vi "Create Keys (AO).vi"(3 "Numeric":i32) -> (1 "AO Keys":string[](array[string]))   [LabVIEW 2016, in "Transport.lvclass"]
uses:
  Transport.lvclass
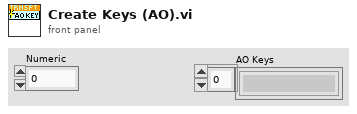
[diagram p1: front panel]
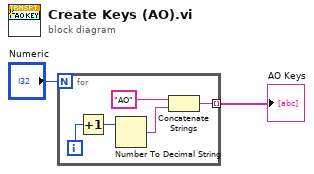
[diagram p0: block diagram]
diagram:
  n1 = for {
    N: "Numeric" -> [_]
    tunnel: [w3] -> w2 mode=indexing
    i -> [w4]
    n2 = Increment(x=w4) -> (x+1=w7:i32)
    n3 = Number To Decimal String(number=w7) -> (decimal integer string=w5:string)  [unwired: 1 in]
    n4 = Concatenate Strings("AO" ("wavenames"), w5) -> (w3:string)
  }
  "AO Keys" <- w2
